vi "rectify_sensor.vi"(6 "Reset":bool, 10 "Configuration":T1, 11 "Array in":sgl[][](array[numeric])=[[0.0, 0.0, 0.0, 0.0]]) -> (3 "Array out":sgl[][](array[numeric]))   [LabVIEW 2013]
uses:
  initialization/configuration.ctl
  initialization/asap_calibration.ctl
  <vilib>/Analysis/Matrix/Datatypes/RealMatrix.ctl
  <vilib>/Analysis/Matrix/NI_Matrix.lvlib
panel:
  out "size(s)":i32[](array[numeric])
  out "Adjustment":sgl[][](array[numeric])
  in  "Enable":bool=TRUE
  # "Each row is the normalized axis positions for one light."
  # "Call at least once with Reset true\nto cache the LUT."
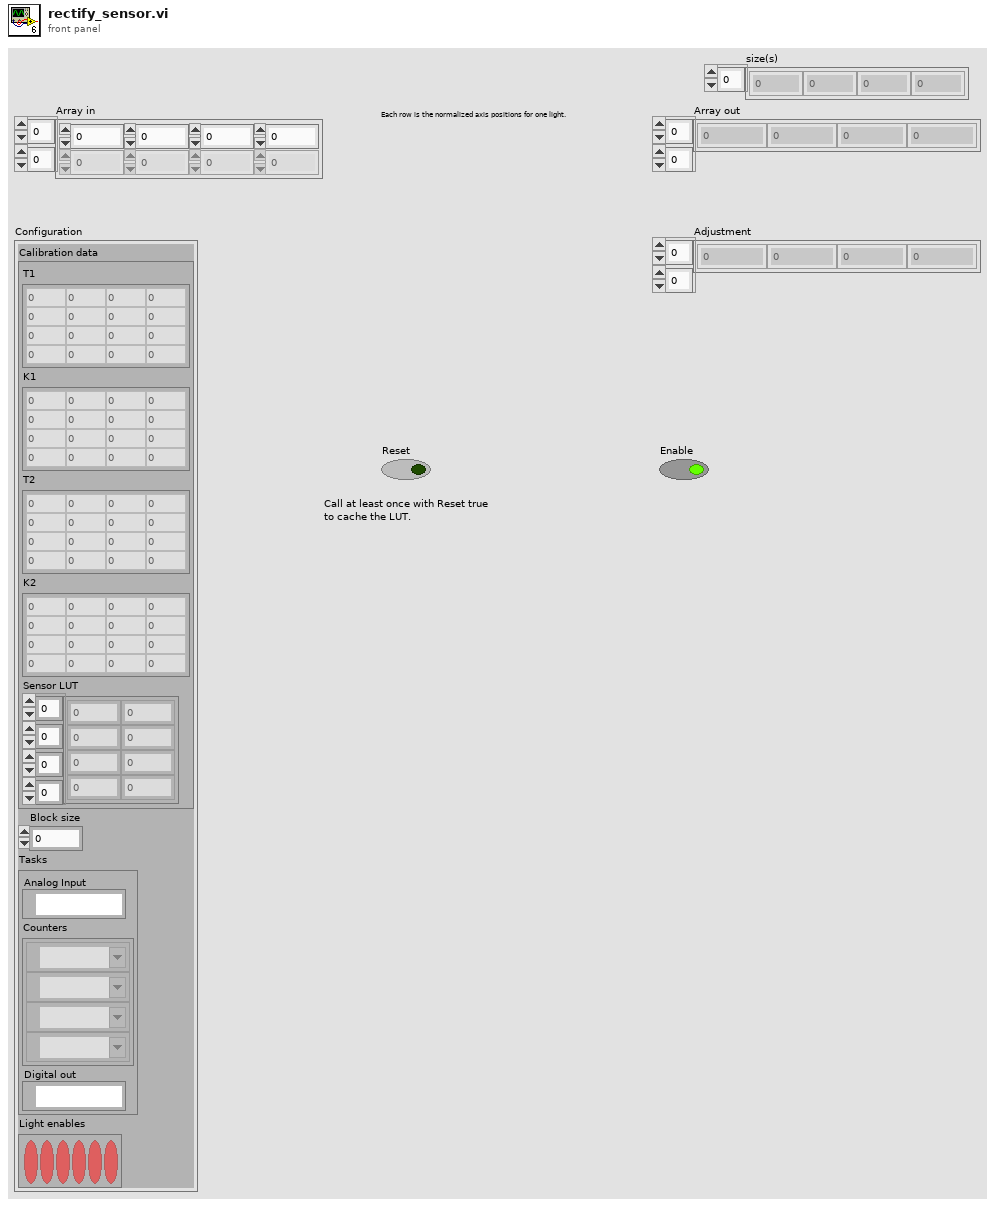
[diagram p1: front panel]
types:
  T1 = typedef "configuration.ctl" = cluster{"Calibration data":T2, "Block size":i32, "Tasks":cluster{"Analog Input":refnum<k21>, "Counters":refnum<k21>[], "Digital out":refnum<k21>}, "Light enables":bool[]}
  T2 = typedef "asap_calibration.ctl" = cluster{"T1":T3, "K1":T3, "T2":T3, "K2":T3, "Sensor LUT":sgl[][][][]}
  T3 = typedef "NI_Matrix.lvlib/RealMatrix.ctl" = dbl[][]
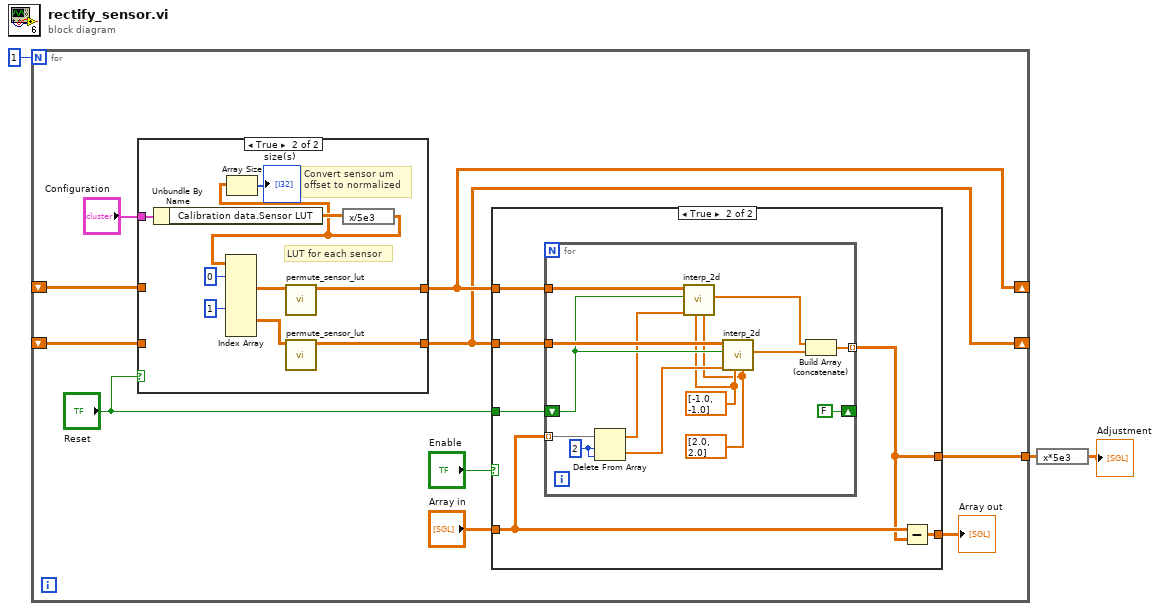
[diagram p0: block diagram]
diagram:
  n1 = for {
    N: 1 -> [_]
    shift-right: [w6] -> _
    shift-left: _ -> [w11]
    shift-right: [w5] -> _
    shift-left: _ -> [w10]
    tunnel: [w4] -> w1
    n2 = case shown="True" "Reset" {
      tunnel: "Configuration" -> [_ w45]
      tunnel: [w35 w43] -> w6
      tunnel: [w34 w39] -> w5
      tunnel: w11 -> [w35 _]
      tunnel: w10 -> [w34 _]
      frame False {
      }
      frame True {
        # "Convert sensor um\noffset to normalized"
        # "LUT for each sensor"
        n3 = Unbundle By Name(w45) -> ("Calibration data.Sensor LUT"=w38:sgl[][][][])
        n4 = expression code="x/5e3"(w38) -> (w37:sgl[][][][])
        n5 = Index Array(array=w37, index (dim 0) #1=0 ("index (vol)"), index (dim 0) #2=1 ("index (vol)")) -> (element #1=w42:sgl[][][], element #2=w41:sgl[][][])  [unwired: 6 in]
        n6 = Array Size(array=w37) -> (size(s)=→"size(s)":i32[])
        n7 = call "permute_sensor_lut.vi"("Sensor LUT in"=w42) -> ("Sensor LUT out"=w43:sgl[][][])  [unwired: 10 in]
        n8 = call "permute_sensor_lut.vi"("Sensor LUT in"=w41) -> ("Sensor LUT out"=w39:sgl[][][])  [unwired: 10 in]
      }
    }
    n9 = case shown="True" "Enable" {
      tunnel: w6 -> [_ w20]
      tunnel: w5 -> [_ w19]
      tunnel: "Reset" -> [_ w18]
      tunnel: [w14 w17] -> w13
      tunnel: "Array in" -> [w14 w16]
      tunnel: [w14 w15] -> w4
      frame False {
      }
      frame True {
        n10 = for {
          tunnel: w20 -> [w33]
          tunnel: w19 -> [w32]
          tunnel: w16 -> [w30] mode=indexing
          tunnel: [w22] -> w15 mode=indexing
          shift-right: [FALSE ("Reset")] -> _
          shift-left: w18 -> [w31]
          w25 = sgl[] [2.0, 2.0] ("Offset")
          w26 = sgl[] [-1.0, -1.0] ("Offset")
          w29 = 2 ("length")
          n11 = Delete From Array(array=w30, length=w29, index=w29) -> (deleted portion=w28:sgl[], array with subset deleted=w27:sgl[])
          n12 = call "interp_2d.vi"("Scale"=w25, "Offset"=w26, "Input x"=w27, "Set LUT"=w31, "Table"=w33) -> ("Output f(x)"=w24:sgl[])  [unwired: 6 in]
          n13 = call "interp_2d.vi"("Scale"=w25, "Offset"=w26, "Input x"=w28, "Set LUT"=w31, "Table"=w32) -> ("Output f(x)"=w23:sgl[])  [unwired: 6 in]
          n14 = Build Array (concatenate)(w24, w23) -> (w22:sgl[])
        }
        n15 = Subtract(x=w16, y=w15) -> (x-y=w17:sgl[][])
      }
    }
    "Array out" <- w13
  }
  n16 = expression code="x*5e3"(w1) -> (→"Adjustment":sgl[][])
